vi "finish communication.vi"(8 "error in (no error)":errorcluster, 11 "Socket in":refnum<class "Socket.lvclass">) -> (0 "error out":errorcluster, 3 "Socket out":refnum<class "Socket.lvclass">)   [LabVIEW 2018, in "Socket.lvclass"]
uses:
  Socket.lvclass
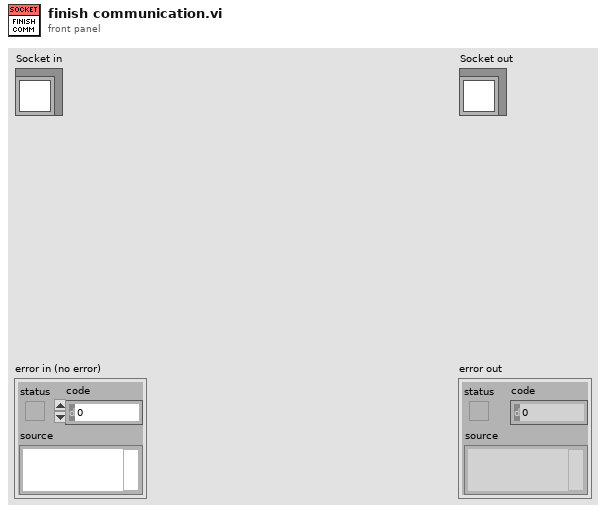
[diagram p1: front panel]
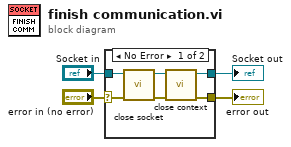
[diagram p0: block diagram]
diagram:
  n1 = case shown="No Error" "error in (no error)" {
    selector: "error in (no error)" -> [w10 w12]
    tunnel: [w8 w12] -> w3
    tunnel: [w5 w11] -> w1
    tunnel: "Socket in" -> [w7 w11]
    frame No Error {
      n2 = call "close socket.vi"("error in (no error)"=w10, "Socket in"=w7) -> ("error out"=w9:errorcluster, "Socket out"=w6:refnum<class "Socket.lvclass">)  [unwired: 8 in]
      n3 = call-dynamic "close context.vi"("error in (no error)"=w9, "Socket in"=w6) -> ("error out"=w8:errorcluster, "Socket out"=w5:refnum<class "Socket.lvclass">)  [unwired: 8 in]
    }
    frame Error {
    }
  }
  "error out" <- w3
  "Socket out" <- w1
